vi "DictionaryTestCopy.vi"() -> ()   [LabVIEW 2017, in "Switch Scripting.lvlib"]
uses:
  Switch Scripting.lvlib
  Routing Channel/Alias Mapping.ctl
  <vilib>/NI Veristand/Custom Device API/Custom Device Channel.ctl
  <vilib>/NI Veristand/Custom Device API/Custom Device Channel Type.ctl
  Shared/Routing and Faulting Custom Device Settings.ctl
  NationalInstruments.VeriStand.SystemDefinitionAPI
  github/niveristand-engine-simulation-toolkit-custom-device/Source/Scripting API/Custom Device/Engine Simulation Toolkit Custom Device Settings.ctl
  <vilib>/NI VeriStand/Custom Device API/Custom Device API.lvlib
  <vilib>/NI Veristand/Custom Device API/Set Item Property (String).vi
  Shared/Switch Shared.lvlib
panel:
  out "All Alias Mappings":T1[](array[typedef])
  out "Alias found":bool
  out "Pin":string
  out "value with bogusName":string[](array[string])
  out "value from GetStringArray":string[](array[string])
  out "new SDF file":path
  in  "Channel":string="RoutingChannel0"
  out "error out":errorcluster
  out "error":string
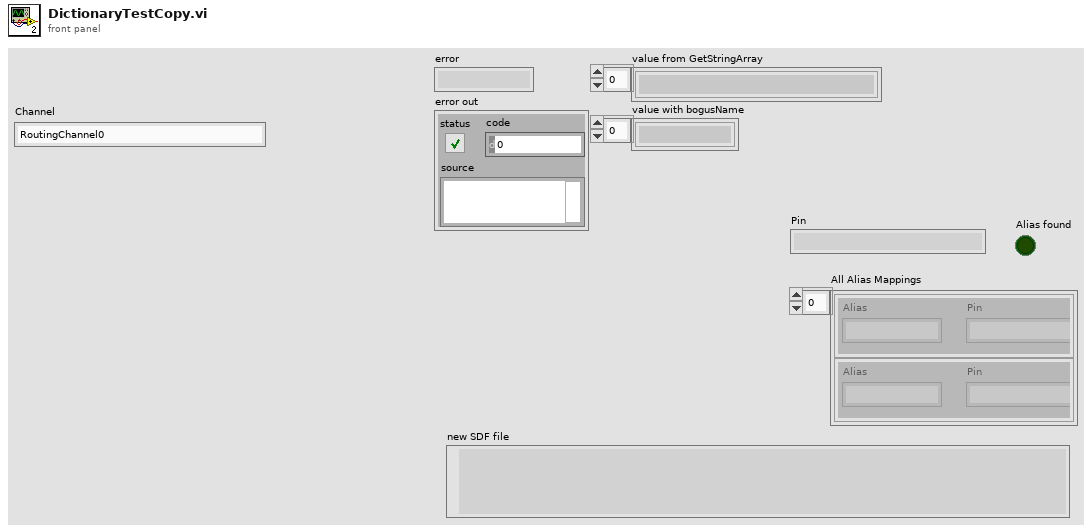
[diagram p1: front panel]
types:
  T1 = typedef "Switch Scripting.lvlib/Alias Mapping.ctl" = cluster{"Alias":string, "Pin":string}
  T2 = typedef "Switch Shared.lvlib/Routing and Faulting Custom Device Settings.ctl" = cluster{"Name":string}
  T3 = typedef "Custom Device API.lvlib/Custom Device Channel.ctl" = cluster{"Type":T4, "Units":string, "Default Value":dbl, "Faultable":bool, "Scalable":bool}
  T4 = typedef "Custom Device API.lvlib/Custom Device Channel Type.ctl" = enum16{"Input", "Output"}
  T5 = typedef "Custom Device API.lvlib/Custom Device Item Ref.ctl" = u64
  T6 = typedef "Engine Simulation Toolkit Scripting API.lvlib/Engine Simulation Toolkit Custom Device Settings.ctl" = cluster{"Name":string, "Execution priority":enum16{"Low", "Medium", "High"}, "Rate decimation":i32, "CPU":i32}
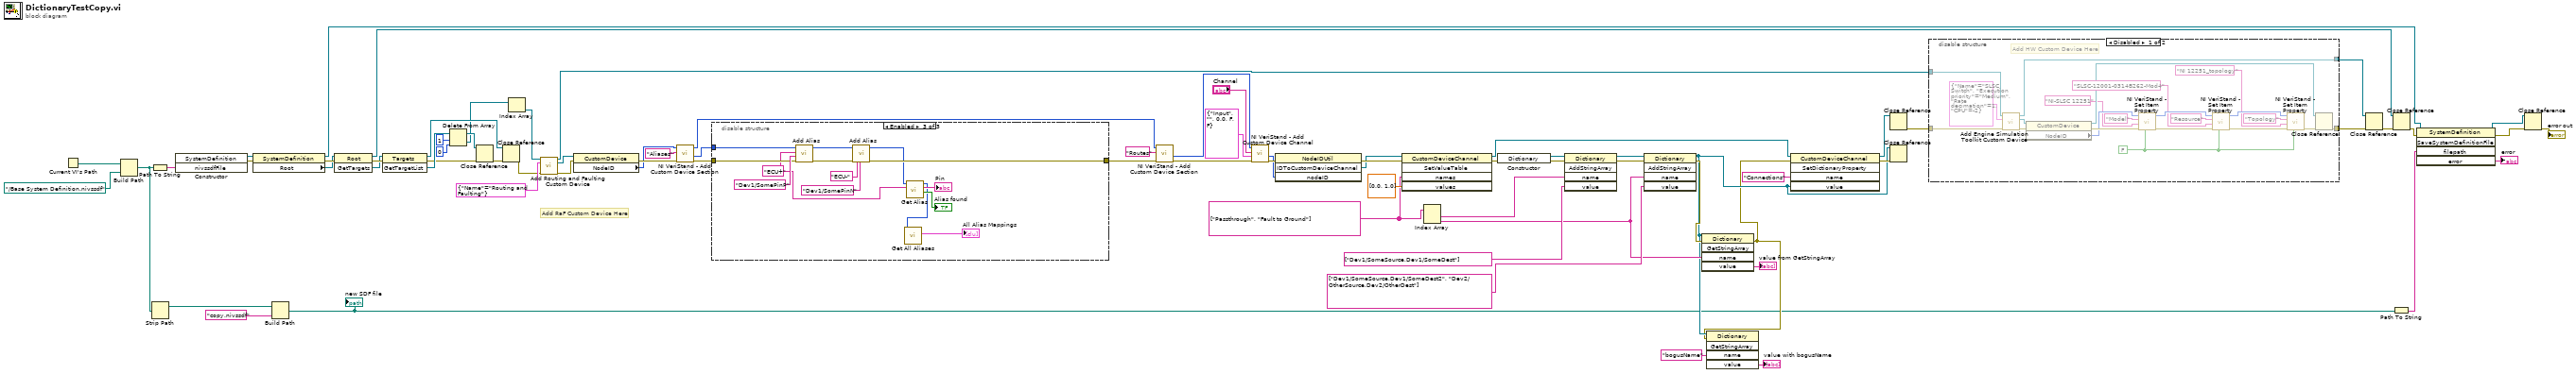
[diagram p0: block diagram]
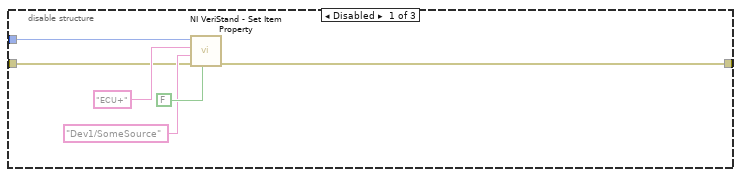
[diagram p2: hidden frame]
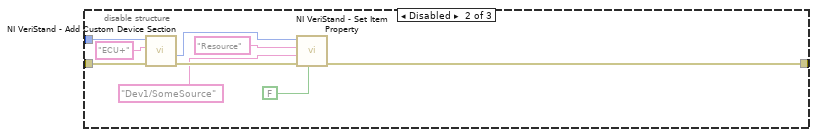
[diagram p3: hidden frame]
diagram:
  w25 = string[] ["Passthrough", "Fault to Ground"] ("names")
  # "Add RaF Custom Device Here"
  n1 = Current VI's Path() -> (path=w19:path)
  n2 = Build Path(base path=w19, name or relative path=path "../Base System Definition.nivssdf" ("Absolute or Relative Path")) -> (appended path=w17:path)
  n3 = Path To String(path=w17) -> (string=w75:string)
  n4 = Strip Path(path=w17) -> (stripped path=w60:path)  [unwired: 1 out]
  n5 = constructor class="SystemDefinition"("nivssdfFile"=w75) -> (reference out=w74:refnum<k24>, error out=w76:errorcluster)  [unwired: 3 in, 2 out]
  n6 = property class="SystemDefinition"(reference=w74, error in=w76) -> (reference out=w61:refnum<k24>, error out=w73:errorcluster, "Root"=w72:refnum<k24>)
  n7 = Build Path(base path=w60, name or relative path="copy.nivssdf") -> (appended path=w2:path)
  "new SDF file" <- w2
  n8 = invoke class="Root" method="GetTargets"(reference=w72, error in=w73) -> (reference out=w57:refnum<k24>, error out=w71:errorcluster, "GetTargets"=w70:refnum<k24>)  [unwired: 1 in]
  n9 = invoke class="Targets" method="GetTargetList"(reference=w70, error in=w71) -> (reference out=w63:refnum<k24>, error out=w66:errorcluster, "GetTargetList"=w69:refnum<k24>[])  [unwired: 1 in]
  n10 = Delete From Array(array=w69, length=1, index=0) -> (deleted portion=w62:refnum<k24>[], array with subset deleted=w65:refnum<k24>[])
  n11 = Close Reference(reference=w65, error in (no error)=w66) -> (error out=w64:errorcluster)
  n12 = Close Reference(reference=w63, error in (no error)=w64) -> (error out=w12:errorcluster)
  n13 = Index Array(array=w62) -> (element=w14:refnum<k24>)  [unwired: 1 in]
  n14 = call "Add Routing and Faulting Custom Device.vi"("Target in"=w14, "Settings"=T2 {"Name"="Routing and Faulting"}, "error in (no error)"=w12) -> ("Target out"=w13:refnum<k24>, "RAF Custom Device"=w10:refnum<k24>, "error out"=w11:errorcluster)  [unwired: 8 in, 2 out]
  n15 = property class="CustomDevice"(reference=w10, error in=w11) -> (error out=w40:errorcluster, "NodeID"=w39:u64)  [unwired: 1 out]
  n16 = call <vilib>:"NI VeriStand - Add Custom Device Section.vi"("error in (no error)"=w40, "Section Name"="Aliases", "Parent Ref in"=w39) -> ("error out"=w33:errorcluster, "Section Ptr"=w32:T5, "Parent Ref out"=w37:T5)  [unwired: 5 in, 1 out]
  n17 = disable-structure shown="Enabled" {
    disable-tunnel: w33 -> [w77 w91 w104]
    disable-tunnel: w32 -> [w78 w90 w101]
    disable-tunnel: [w81 w85 w99] -> w31
    frame Disabled {
      n18 = call-poly <vilib>:"NI VeriStand - Set Item Property.vi"("Binary String (T)"=FALSE, "error in (no error)"=w77, "Value"="Dev1/SomeSource" ("Property Name"), "Property Name"="ECU+", "Item Ref in"=w78) -> ("error out"=w81:errorcluster)  [unwired: 4 in, 2 out]
    }
    frame Disabled {
      n19 = call <vilib>:"NI VeriStand - Add Custom Device Section.vi"("error in (no error)"=w91, "Section Name"="ECU+", "Parent Ref in"=w90) -> ("error out"=w88:errorcluster, "Section Ptr"=w87:T5)  [unwired: 5 in, 2 out]
      n20 = call-poly <vilib>:"NI VeriStand - Set Item Property.vi"("Binary String (T)"=FALSE, "error in (no error)"=w88, "Value"="Dev1/SomeSource" ("Property Name"), "Property Name"="Resource", "Item Ref in"=w87) -> ("error out"=w85:errorcluster)  [unwired: 4 in, 2 out]
    }
    frame Enabled {
      w96 = "ECU+" ("Property Name")
      n21 = call "Add Alias.vi"("error in (no error)"=w104, "Pin"="Dev1/SomePinP" ("Property Name"), "Alias"=w96, "Aliases Section Ptr in"=w101) -> ("error out"=w97:errorcluster, "Aliases Section Ptr out"=w98:T5)  [unwired: 6 in]
      n22 = call "Add Alias.vi"("error in (no error)"=w97, "Pin"="Dev1/SomePinN" ("Property Name"), "Alias"="ECU-" ("Property Name"), "Aliases Section Ptr in"=w98) -> ("error out"=w99:errorcluster, "Aliases Section Ptr out"=w93:T5)  [unwired: 6 in]
      n23 = call "Get Alias.vi"("Alias"=w96, "Aliases Section Ptr in"=w93) -> ("Alias found"=→"Alias found":bool, "Pin"=→"Pin":string, "Aliases Section Ptr out"=w92:T5)  [unwired: 6 in, 1 out]
      n24 = call "Get All Aliases.vi"("Aliases Section Ptr in"=w92) -> ("All Alias Mappings"=→"All Alias Mappings":T1[])  [unwired: 7 in, 3 out]
    }
  }
  n25 = call <vilib>:"NI VeriStand - Add Custom Device Section.vi"("error in (no error)"=w31, "Section Name"="Routes", "Parent Ref in"=w37) -> ("error out"=w35:errorcluster, "Section Ptr"=w34:T5)  [unwired: 5 in, 2 out]
  n26 = call <vilib>:"NI VeriStand - Add Custom Device Channel.vi"("error in (no error)"=w35, "Channel"=T3 {"Type"=enum."Input", "Units"="", "Default Value"=0.0, "Faultable"=FALSE, "Scalable"=FALSE}, "Channel Name"="Channel", "Parent Ref in"=w34) -> ("error out"=w42:errorcluster, "Channel Ref"=w41:T5)  [unwired: 4 in, 2 out]
  n27 = invoke class="NodeIDUtil" method="IDToCustomDeviceChannel"(error in=w42, "nodeID"=w41) -> (error out=w45:errorcluster, "IDToCustomDeviceChannel"=w1:refnum<k24>)  [unwired: 2 in, 2 out]
  n28 = invoke class="CustomDeviceChannel" method="SetValueTable"(reference=w1, error in=w45, "names"=w25, "values"=dbl[] [0.0, 1.0]) -> (reference out=w44:refnum<k24>, error out=w43:errorcluster)  [unwired: 1 in, 3 out]
  n29 = Index Array(array=w25) -> (element #1=w24:string, element #2=w9:string)  [unwired: 2 in]
  n30 = constructor class="Dictionary"(error in=w43) -> (reference out=w50:refnum<k24>, error out=w51:errorcluster)  [unwired: 2 in, 1 out]
  n31 = invoke class="Dictionary" method="AddStringArray"(reference=w50, error in=w51, "name"=w24, "value"=string[] ["Dev1/SomeSource,Dev1/SomeDest"]) -> (reference out=w21:refnum<k24>, error out=w22:errorcluster)  [unwired: 1 in, 3 out]
  n32 = invoke class="Dictionary" method="AddStringArray"(reference=w21, error in=w22, "name"=w9, "value"=string[] ["Dev1/SomeSource,Dev1/SomeDest2", "Dev2/OtherSource,Dev2/OtherDest"]) -> (reference out=w6:refnum<k24>, error out=w7:errorcluster)  [unwired: 1 in, 3 out]
  n33 = invoke class="Dictionary" method="GetStringArray"(reference=w6, error in=w7, "name"=w9) -> (error out=w3:errorcluster, "value"=→"value from GetStringArray":string[])  [unwired: 2 in, 3 out]
  n34 = invoke class="Dictionary" method="GetStringArray"(reference=w6, error in=w3, "name"="bogusName") -> ("value"=→"value with bogusName":string[])  [unwired: 2 in, 4 out]
  n35 = invoke class="CustomDeviceChannel" method="SetDictionaryProperty"(reference=w44, error in=w3, "name"="Connections", "value"=w6) -> (reference out=w49:refnum<k24>, error out=w47:errorcluster)  [unwired: 1 in, 3 out]
  n36 = Close Reference(reference=w49) -> (error out=w30:errorcluster)  [unwired: 1 in]
  n37 = Close Reference(reference=w6, error in (no error)=w47) -> ()  [unwired: 1 out]
  n38 = disable-structure shown="Disabled" {
    disable-tunnel: w30 -> [w127 w128]
    disable-tunnel: w13 -> [w126 w129]
    disable-tunnel: [w115 w128] -> w29
    disable-tunnel: [w106 w129] -> w16
    frame Disabled {
      w119 = FALSE ("Binary String (T)")
      # "Add HW Custom Device Here"
      n39 = call "Add Engine Simulation Toolkit Custom Device.vi"("error in (no error)"=w127, "Settings"=T6 {"Name"="SLSC Switch", "Execution priority"=enum."Medium", "Rate decimation"=1, "CPU"=-2}, "Target in"=w126) -> ("error out"=w124:errorcluster, "EST Custom Device"=w123:refnum<k24>, "Target out"=w106:refnum<k24>)  [unwired: 6 in]
      n40 = property class="CustomDevice"(reference=w123, error in=w124) -> (reference out=w114:refnum<k24>, error out=w122:errorcluster, "NodeID"=w121:u64)
      n41 = call-poly <vilib>:"NI VeriStand - Set Item Property.vi"("Binary String (T)"=w119, "error in (no error)"=w122, "Value"="NI-SLSC 12251", "Property Name"="Model", "Item Ref in"=w121) -> ("error out"=w118:errorcluster, "Item Ref out"=w113:T5)  [unwired: 4 in, 1 out]
      n42 = call-poly <vilib>:"NI VeriStand - Set Item Property.vi"("Binary String (T)"=w119, "error in (no error)"=w118, "Value"="SLSC-12001-0314B262-Mod4", "Property Name"="Resource", "Item Ref in"=w113) -> ("error out"=w117:errorcluster, "Item Ref out"=w112:T5)  [unwired: 4 in, 1 out]
      n43 = call-poly <vilib>:"NI VeriStand - Set Item Property.vi"("Binary String (T)"=w119, "error in (no error)"=w117, "Value"="NI 12251_topology", "Property Name"="Topology", "Item Ref in"=w112) -> ("error out"=w116:errorcluster)  [unwired: 4 in, 2 out]
      n44 = Close Reference(reference=w114, error in (no error)=w116) -> (error out=w115:errorcluster)
    }
    frame Enabled {
    }
  }
  n45 = Close Reference(reference=w16, error in (no error)=w29) -> (error out=w28:errorcluster)
  n46 = Path To String(path=w2) -> (string=w58:string)
  n47 = Close Reference(reference=w57, error in (no error)=w28) -> (error out=w27:errorcluster)
  n48 = invoke class="SystemDefinition" method="SaveSystemDefinitionFile"(reference=w61, error in=w27, "filepath"=w58) -> (reference out=w56:refnum<k24>, error out=w26:errorcluster, "error"=→"error":string)  [unwired: 2 in, 2 out]
  n49 = Close Reference(reference=w56, error in (no error)=w26) -> (error out=→"error out":errorcluster)
